vi "mqttCmdCreate.vi"(8 "error in (no error)":errorcluster) -> (0 "error out":errorcluster, 3 "mqttCmdPingResponse out":refnum<class "mqttCmdPingResponse.lvclass">)   [LabVIEW 2020, in "mqttCmdPingResponse.lvclass"]
uses:
  mqttCmdPingResponse.lvclass
  C:/Projects/Libraries/Gore SM 2020/mqtt-LabVIEW/src/class/mqtt/mqttCmd/mqttCmd.lvclass
  mqttTypedef/mqttMessageType.ctl
  mqttTypedef/mqttQOSlevel.ctl
  mqttCmd.lvclass/mqttCmd.ctl
  Properties/Write Datagram.vi
  mqttCmd.lvclass
  mqtt.lvclass
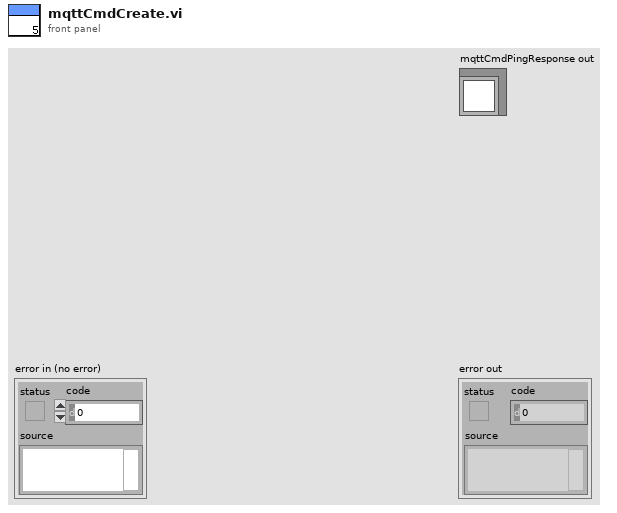
[diagram p1: front panel]
types:
  T1 = typedef "mqtt.lvclass/mqttQOSlevel.ctl" = enum8{"At most once", "At least once", "Exactly once", "Reserved"}
  T2 = typedef "mqtt.lvclass/mqttMessageType.ctl" = enum32{"Reserved", "CONNECT", "CONNACK", "PUBLISH", "PUBACK", "PUBREC", "PUBREL", "PUBCOMP", "SUBSCRIBE", "SUBACK", "UNSUBSCRIBE", "UNSUBACK", "PINGREQ", "PINGRESP", "DISCONNECT", "Reserved2"}
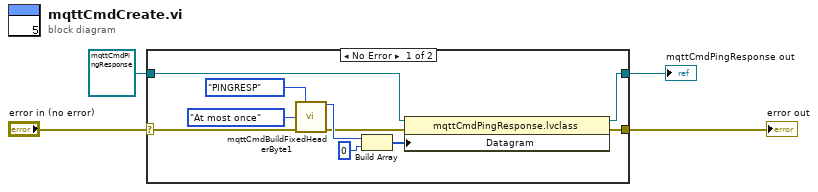
[diagram p0: block diagram]
diagram:
  n1 = case shown="No Error" "error in (no error)" {
    selector: "error in (no error)" -> [w10 w16]
    tunnel: [w5 w16] -> w3
    tunnel: [w8 w15] -> w1
    tunnel: refnum<class "mqttCmdPingResponse.lvclass"> refnum ("mqttCmdPingResponse in") -> [w9 w15]
    frame No Error {
      n2 = call "mqttCmdBuildFixedHeaderByte1.vi"("MessageType"=mqttMessageType."PINGRESP", "QoS (At most once)"=mqttQOSlevel."At most once", "error in (no error)"=w10) -> ("byte1"=w12:u8, "error out"=w7:errorcluster)  [unwired: 11 in]
      n3 = Build Array(w12, u8 0 ("byte1")) -> (w6:u8[])
      n4 = property class="mqttCmdPingResponse.lvclass"(reference=w9, error in=w7, "Datagram"=w6) -> (reference out=w8:refnum<class "mqttCmdPingResponse.lvclass">, error out=w5:errorcluster)
    }
    frame Error {
    }
  }
  "error out" <- w3
  "mqttCmdPingResponse out" <- w1
